vi "App_Main Release.vi"(8 "error in":errorcluster) -> (0 "error out":errorcluster)   [LabVIEW 2015, in "Application 2.lvlib"]
uses:
  Application 2.lvlib
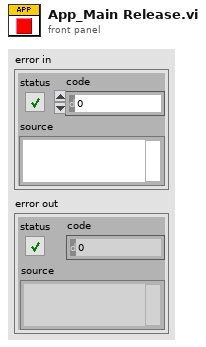
[diagram p1: front panel]
types:
  T1 = typedef "Application 2.lvlib/App_Main Data.ctl" = cluster{"VI Refnum":refnum<vi>, "Subpanel":refnum<vi>, "Connection ID":refnum<k5>, "Meta data":T2[], "Main Queue":T4, "User Data":T5}
  T2 = typedef "stm_MetaElement.ctl" = cluster{"Name":T3}
  T3 = typedef "stm_MetaDataElement.ctl" = string
  T4 = typedef "Application 2.lvlib/App_Main Queue.ctl" = cluster{"Main Loop Queue":refnum<queue>}
  T5 = typedef "User Data.ctl" = cluster{"Name":string, "Email":string, "Phone Number":string, "User Picture":u32[][], "Last Login Time":timestamp}
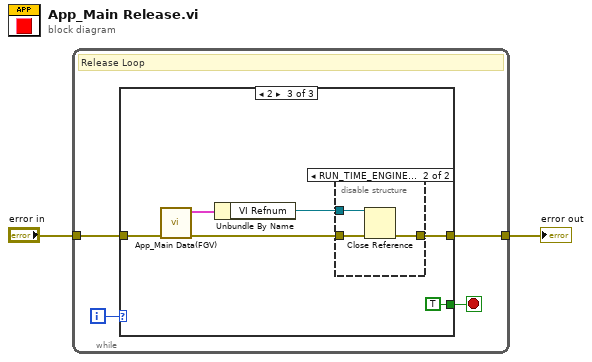
[diagram p0: block diagram]
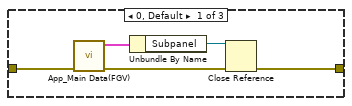
[diagram p2: hidden frame]
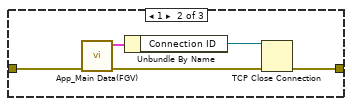
[diagram p3: hidden frame]
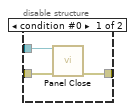
[diagram p4: hidden frame]
diagram:
  n1 = while {
    tunnel: "error in" -> [w5]
    tunnel: [w4] -> w1
    i -> [w6]
    stop <- w3 stop-if-true
    # "Release Loop"
    n2 = case shown="2" w6 {
      tunnel: w5 -> [w11 w16 w22]
      tunnel: [w7 w12 w18] -> w4
      tunnel: [_ _ TRUE] -> w3
      frame 0, Default {
        n3 = call "App_Main Data(FGV).vi"("error in"=w11) -> ("error out"=w9:errorcluster, "Main Data Out"=w10:T1)  [unwired: 9 in]
        n4 = Unbundle By Name(w10) -> ("Subpanel"=w8:refnum<vi>)
        n5 = Close Reference(reference=w8, error in (no error)=w9) -> (error out=w7:errorcluster)
      }
      frame 1 {
        n6 = call "App_Main Data(FGV).vi"("error in"=w16) -> ("error out"=w14:errorcluster, "Main Data Out"=w15:T1)  [unwired: 9 in]
        n7 = Unbundle By Name(w15) -> ("Connection ID"=w13:refnum<k5>)
        n8 = TCP Close Connection(connection ID=w13, error in (no error)=w14) -> (error out=w12:errorcluster)  [unwired: 1 in, 1 out]
      }
      frame 2 {
        n9 = call "App_Main Data(FGV).vi"("error in"=w22) -> ("error out"=w20:errorcluster, "Main Data Out"=w21:T1)  [unwired: 9 in]
        n10 = Unbundle By Name(w21) -> ("VI Refnum"=w19:refnum<vi>)
        n11 = disable-structure shown="RUN_TIME_ENGINE==False" {
          disable-tunnel: w20 -> [w25 w27]
          disable-tunnel: [w24 w28] -> w18
          disable-tunnel: w19 -> [w23 w26]
          frame condition #0 {
            n12 = call "Panel Close.vi"("error in"=w25, "VI Reference"=w23) -> ("error out"=w24:errorcluster)  [unwired: 9 in]
          }
          frame condition #1 (active) {
            n13 = Close Reference(reference=w26, error in (no error)=w27) -> (error out=w28:errorcluster)
          }
        }
      }
    }
  }
  "error out" <- w1
